vi "Traffic_Light_Simulation (1).vi"() -> ()   [LabVIEW 2020]
panel:
  out "Green 13":bool
  out "Green 11":bool
  out "Green 14":bool
  out "Green 12":bool
  out "Green 10":bool
  out "Green 9":bool
  out "Green 8":bool
  out "Green 7":bool
  out "Boolean 3":bool
  out "Yellow5":bool
  out "Green 6":bool
  out "Red 6":bool
  out "Boolean":bool
  out "Boolean 5":bool
  out "Boolean 4":bool
  out "Boolean 2":bool
  out "Red 5":bool
  out "Green 5":bool
  out "Yellow 4":bool
  out "Green 4":bool
  out "Red 4":bool
  out "Yellow4":bool
  out "Yellow 3":bool
  out "Green 3":bool
  out "Red 3":bool
  out "Red 2":bool
  out "Yellow 2":bool
  out "Green 2":bool
  in  "stop":bool
  # "|\n|\n|\n|\n|\n|\n|\n|\n|\n|\n|"
  # "Pedesterian Signal"
  # "Pedesterian Signal"
  # "Zebra Crossing"
  # "| | | | | | | | | | | | | | | | | | | | | | | | | | | | | |"
  # "Left Light"
  # "| |\n| |\n| |\n| |\n| |\n| |\n| |\n| |\n| |\n| |\n| |"
  # "| |\n| |\n| |\n| |\n| |\n| |\n| |\n| |\n| |\n| |\n| |"
  # "Left Light"
  # "Left Light"
  # "----------------------------------"
  # "Traffic Light Simulation"
  # "----------------------------------"
  # "Left Light"
  # "|\n|\n|\n|\n|\n|\n|\n|\n|\n|\n|"
  # "| | | | | | | | | | | | | | | | | | | | | | | | | | | | | |"
  # "Pedesterian Signal"
  # "Pedesterian Signal"
  # "Meaning of Traffic Lights"
  # "Go"
  # "Ready to Stop"
  # "Stop"
  # "Only Left Turns"
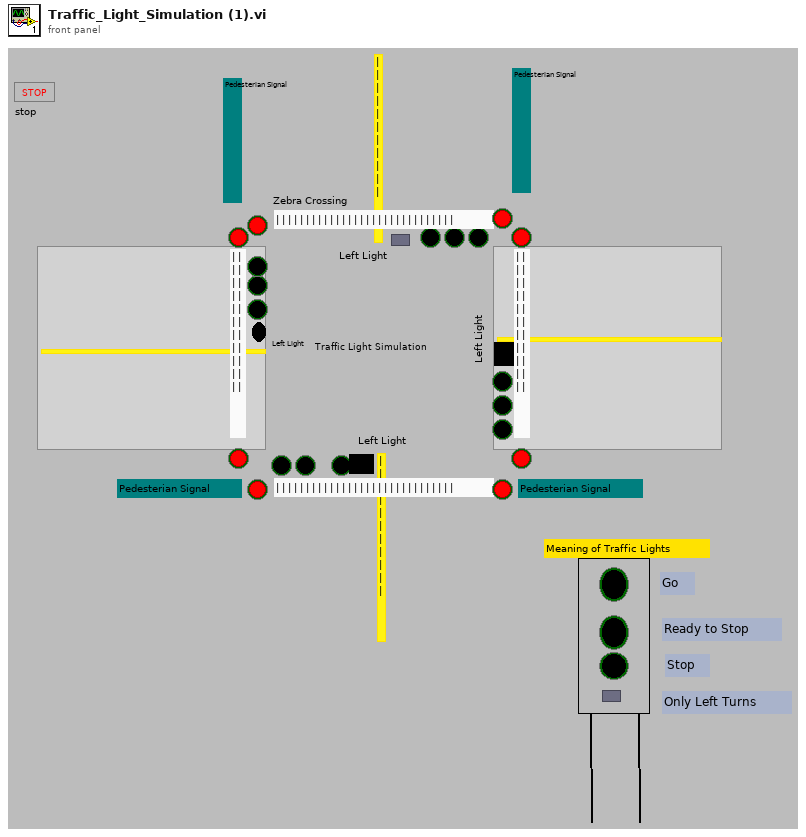
[diagram p1: front panel]
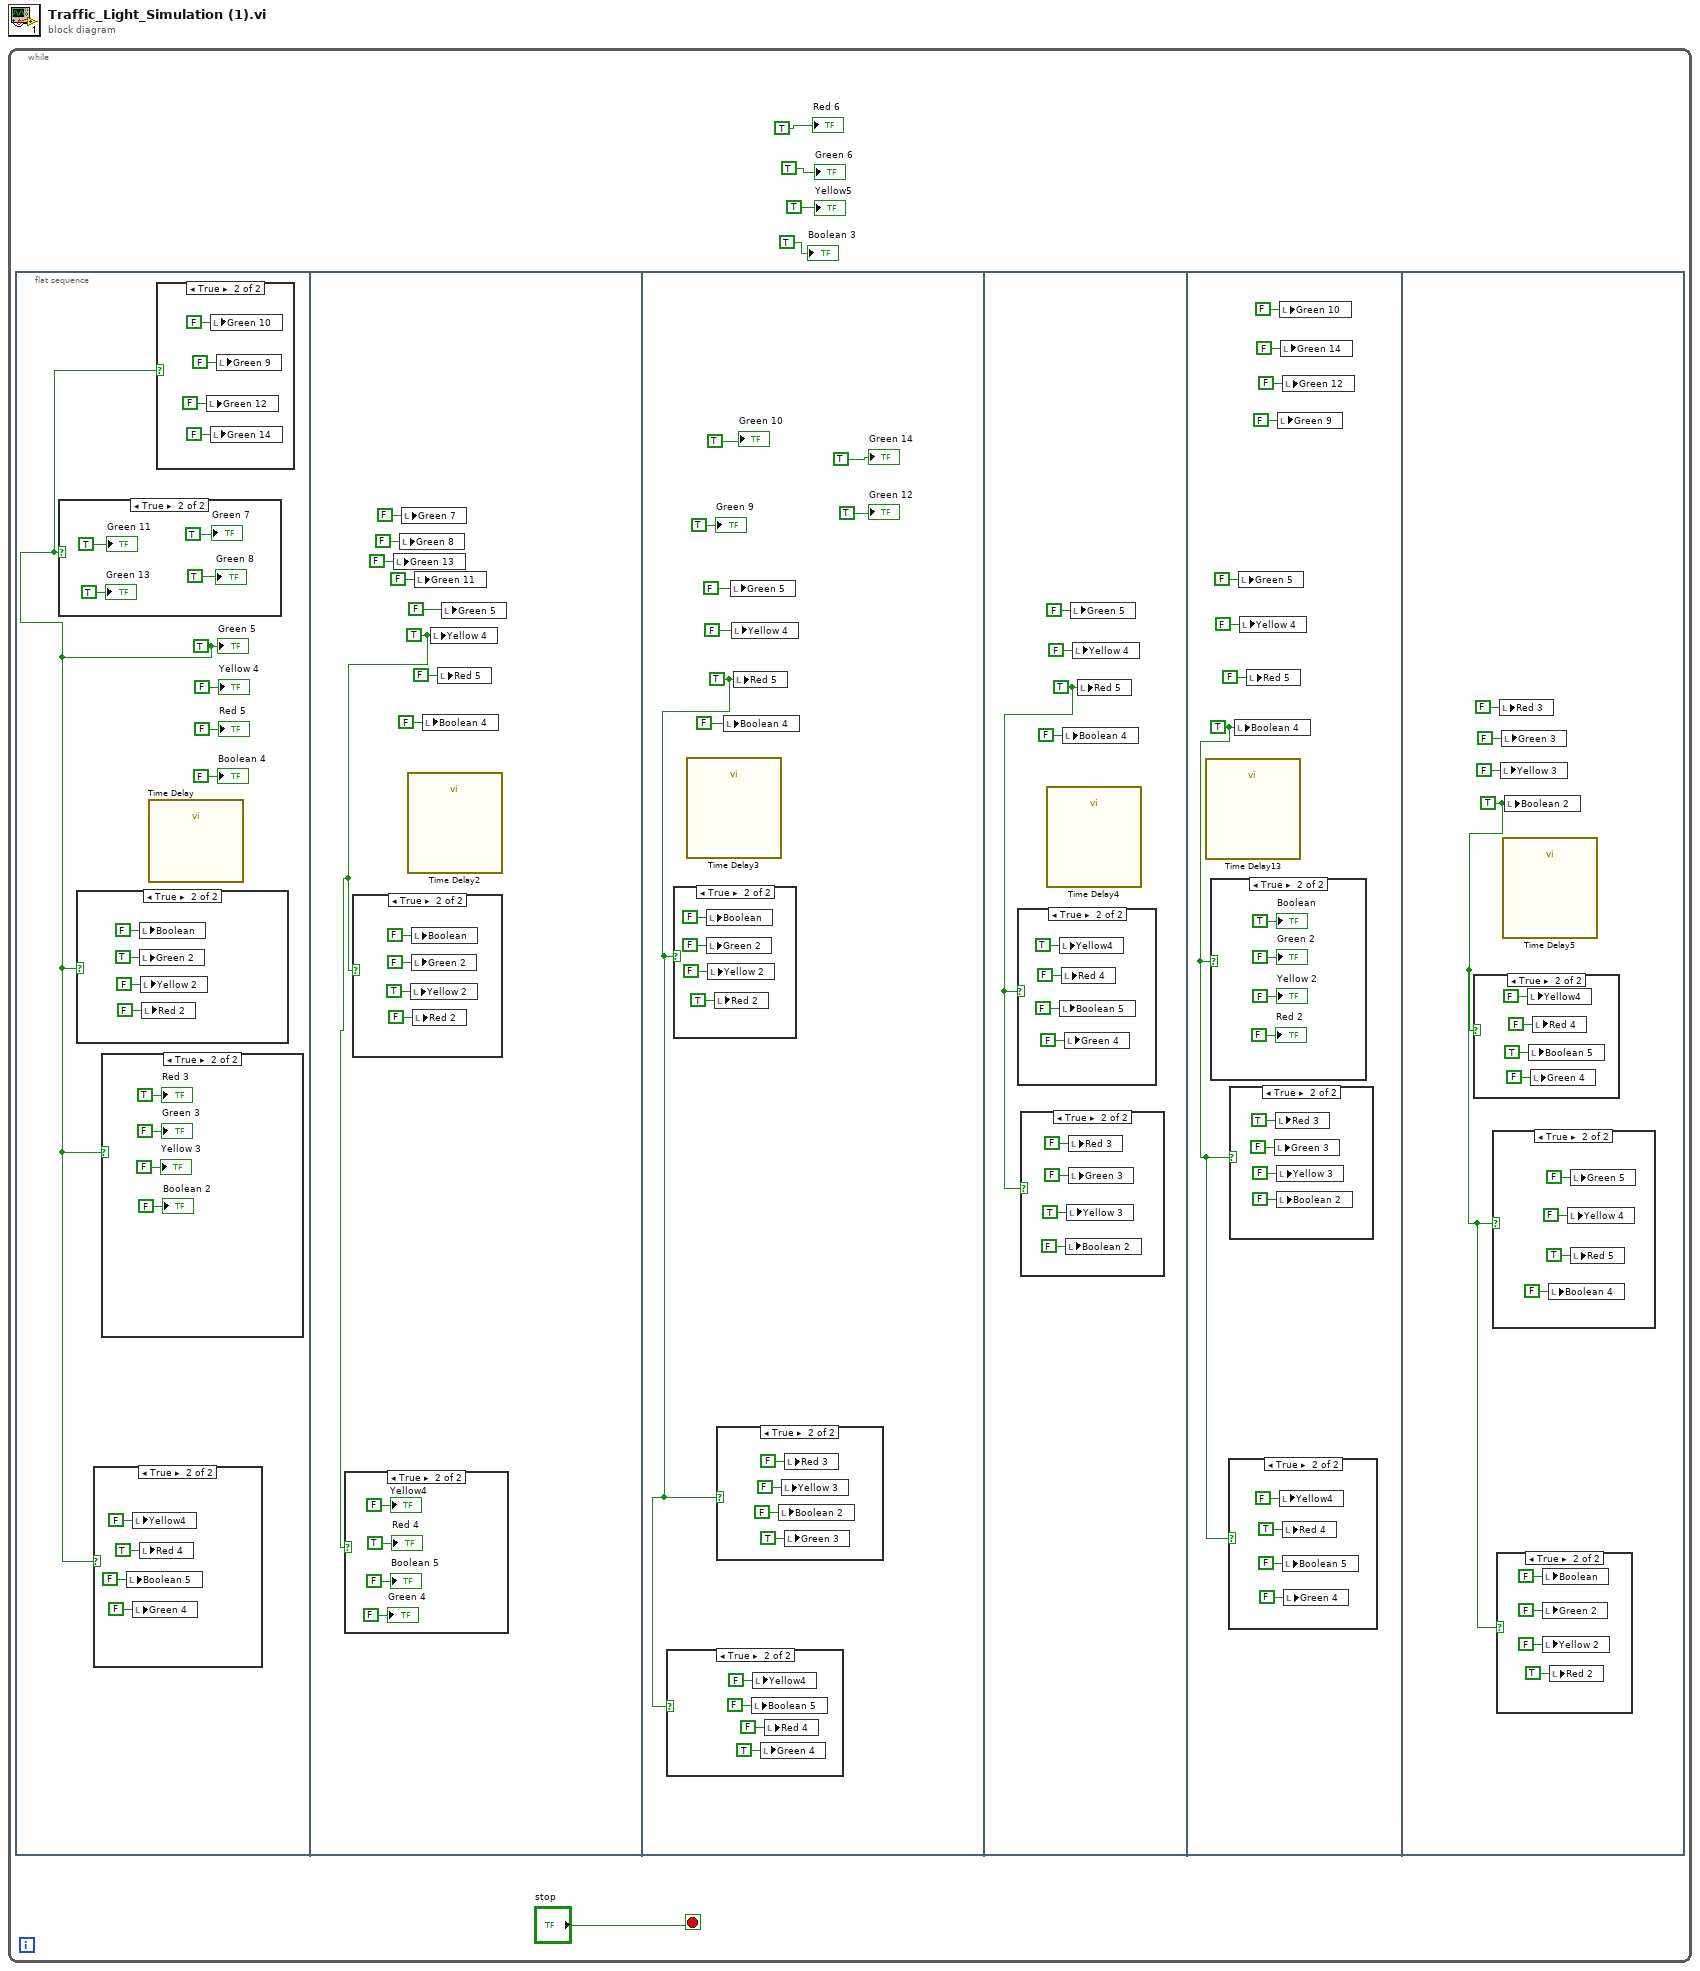
[diagram p0: block diagram]
diagram:
  n1 = while {
    stop <- "stop" stop-if-true
    n2 = flat-sequence {
      frame #0 {
        w6 = TRUE ("Green 5")
        n3 = case shown="True" w6 {
          frame False {
          }
          frame True {
            "Green 7" <- TRUE ("Green 7")
            "Green 11" <- TRUE ("Green 11")
            "Green 13" <- TRUE ("Green 13")
            "Green 8" <- TRUE ("Green 8")
          }
        }
        n4 = case shown="True" w6 {
          frame False {
          }
          frame True {
            n5 = local write "Boolean"(FALSE ("Boolean")) -> ()
            n6 = local write "Green 2"(TRUE ("Green 2")) -> ()
            n7 = local write "Yellow 2"(FALSE ("Yellow 2")) -> ()
            n8 = local write "Red 2"(FALSE ("Red 2")) -> ()
          }
        }
        n9 = case shown="True" w6 {
          frame False {
          }
          frame True {
            n10 = local write "Boolean 5"(FALSE ("Boolean 5")) -> ()
            n11 = local write "Yellow4"(FALSE ("Yellow4")) -> ()
            n12 = local write "Green 4"(FALSE ("Green 4")) -> ()
            n13 = local write "Red 4"(TRUE ("Red 4")) -> ()
          }
        }
        n14 = case shown="True" w6 {
          frame False {
          }
          frame True {
            "Red 3" <- TRUE ("Red 3")
            "Green 3" <- FALSE ("Green 3")
            "Yellow 3" <- FALSE ("Yellow 3")
            "Boolean 2" <- FALSE ("Boolean 2")
          }
        }
        n15 = call "Time Delay"() -> ()  [unwired: 11 in, 1 out]
        n16 = case shown="True" w6 {
          frame False {
          }
          frame True {
            n17 = local write "Green 12"(FALSE ("Green 12")) -> ()
            n18 = local write "Green 10"(FALSE ("Green 10")) -> ()
            n19 = local write "Green 14"(FALSE ("Green 14")) -> ()
            n20 = local write "Green 9"(FALSE ("Green 9")) -> ()
          }
        }
        "Yellow 4" <- FALSE ("Yellow 4")
        "Green 5" <- w6
        "Red 5" <- FALSE ("Red 5")
        "Boolean 4" <- FALSE ("Boolean 4")
      }
      frame #1 {
        w34 = TRUE ("Yellow 4")
        n21 = case shown="True" w34 {
          frame False {
          }
          frame True {
            "Yellow4" <- FALSE ("Yellow4")
            "Red 4" <- TRUE ("Red 4")
            "Boolean 5" <- FALSE ("Boolean 5")
            "Green 4" <- FALSE ("Green 4")
          }
        }
        n22 = case shown="True" w34 {
          frame False {
          }
          frame True {
            n23 = local write "Yellow 2"(TRUE ("Yellow 2")) -> ()
            n24 = local write "Boolean"(FALSE ("Boolean")) -> ()
            n25 = local write "Green 2"(FALSE ("Green 2")) -> ()
            n26 = local write "Red 2"(FALSE ("Red 2")) -> ()
          }
        }
        n27 = local write "Green 13"(FALSE ("Green 13")) -> ()
        n28 = local write "Green 8"(FALSE ("Green 8")) -> ()
        n29 = local write "Green 7"(FALSE ("Green 7")) -> ()
        n30 = call "Time Delay2"() -> ()  [unwired: 11 in, 1 out]
        n31 = local write "Green 11"(FALSE ("Green 11")) -> ()
        n32 = local write "Boolean 4"(FALSE ("Boolean 4")) -> ()
        n33 = local write "Yellow 4"(w34) -> ()
        n34 = local write "Red 5"(FALSE ("Red 5")) -> ()
        n35 = local write "Green 5"(FALSE ("Green 5")) -> ()
      }
      frame #2 {
        w50 = TRUE ("Red 5")
        n36 = case shown="True" w50 {
          frame False {
          }
          frame True {
            n37 = local write "Boolean 5"(FALSE ("Boolean 5")) -> ()
            n38 = local write "Yellow4"(FALSE ("Yellow4")) -> ()
            n39 = local write "Green 4"(TRUE ("Green 4")) -> ()
            n40 = local write "Red 4"(FALSE ("Red 4")) -> ()
          }
        }
        n41 = case shown="True" w50 {
          frame False {
          }
          frame True {
            n42 = local write "Boolean"(FALSE ("Boolean")) -> ()
            n43 = local write "Green 2"(FALSE ("Green 2")) -> ()
            n44 = local write "Yellow 2"(FALSE ("Yellow 2")) -> ()
            n45 = local write "Red 2"(TRUE ("Red 2")) -> ()
          }
        }
        n46 = call "Time Delay3"() -> ()  [unwired: 11 in, 1 out]
        n47 = case shown="True" w50 {
          frame False {
          }
          frame True {
            n48 = local write "Boolean 2"(FALSE ("Boolean 2")) -> ()
            n49 = local write "Yellow 3"(FALSE ("Yellow 3")) -> ()
            n50 = local write "Red 3"(FALSE ("Red 3")) -> ()
            n51 = local write "Green 3"(TRUE ("Green 3")) -> ()
          }
        }
        n52 = local write "Boolean 4"(FALSE ("Boolean 4")) -> ()
        n53 = local write "Green 5"(FALSE ("Green 5")) -> ()
        n54 = local write "Yellow 4"(FALSE ("Yellow 4")) -> ()
        n55 = local write "Red 5"(w50) -> ()
        "Green 14" <- TRUE ("Green 14")
        "Green 10" <- TRUE ("Green 10")
        "Green 9" <- TRUE ("Green 9")
        "Green 12" <- TRUE ("Green 12")
      }
      frame #3 {
        w66 = TRUE ("Red 5")
        n56 = case shown="True" w66 {
          frame False {
          }
          frame True {
            n57 = local write "Yellow4"(TRUE ("Yellow4")) -> ()
            n58 = local write "Boolean 5"(FALSE ("Boolean 5")) -> ()
            n59 = local write "Red 4"(FALSE ("Red 4")) -> ()
            n60 = local write "Green 4"(FALSE ("Green 4")) -> ()
          }
        }
        n61 = case shown="True" w66 {
          frame False {
          }
          frame True {
            n62 = local write "Boolean 2"(FALSE ("Boolean 2")) -> ()
            n63 = local write "Yellow 3"(TRUE ("Yellow 3")) -> ()
            n64 = local write "Red 3"(FALSE ("Red 3")) -> ()
            n65 = local write "Green 3"(FALSE ("Green 3")) -> ()
          }
        }
        n66 = call "Time Delay4"() -> ()  [unwired: 11 in, 1 out]
        n67 = local write "Boolean 4"(FALSE ("Boolean 4")) -> ()
        n68 = local write "Green 5"(FALSE ("Green 5")) -> ()
        n69 = local write "Yellow 4"(FALSE ("Yellow 4")) -> ()
        n70 = local write "Red 5"(w66) -> ()
      }
      frame #4 {
        w82 = TRUE ("Boolean 4")
        n71 = call "Time Delay13"() -> ()  [unwired: 11 in, 1 out]
        n72 = case shown="True" w82 {
          frame False {
          }
          frame True {
            "Boolean" <- TRUE ("Boolean")
            "Green 2" <- FALSE ("Green 2")
            "Red 2" <- FALSE ("Red 2")
            "Yellow 2" <- FALSE ("Yellow 2")
          }
        }
        n73 = case shown="True" w82 {
          frame False {
          }
          frame True {
            n74 = local write "Yellow4"(FALSE ("Yellow4")) -> ()
            n75 = local write "Red 4"(TRUE ("Red 4")) -> ()
            n76 = local write "Boolean 5"(FALSE ("Boolean 5")) -> ()
            n77 = local write "Green 4"(FALSE ("Green 4")) -> ()
          }
        }
        n78 = case shown="True" w82 {
          frame False {
          }
          frame True {
            n79 = local write "Green 3"(FALSE ("Green 3")) -> ()
            n80 = local write "Red 3"(TRUE ("Red 3")) -> ()
            n81 = local write "Yellow 3"(FALSE ("Yellow 3")) -> ()
            n82 = local write "Boolean 2"(FALSE ("Boolean 2")) -> ()
          }
        }
        n83 = local write "Boolean 4"(w82) -> ()
        n84 = local write "Green 5"(FALSE ("Green 5")) -> ()
        n85 = local write "Yellow 4"(FALSE ("Yellow 4")) -> ()
        n86 = local write "Red 5"(FALSE ("Red 5")) -> ()
        n87 = local write "Green 9"(FALSE ("Green 9")) -> ()
        n88 = local write "Green 10"(FALSE ("Green 10")) -> ()
        n89 = local write "Green 14"(FALSE ("Green 14")) -> ()
        n90 = local write "Green 12"(FALSE ("Green 12")) -> ()
      }
      frame #5 {
        w98 = TRUE ("Boolean 2")
        n91 = case shown="True" w98 {
          frame False {
          }
          frame True {
            n92 = local write "Yellow4"(FALSE ("Yellow4")) -> ()
            n93 = local write "Boolean 5"(TRUE ("Boolean 5")) -> ()
            n94 = local write "Green 4"(FALSE ("Green 4")) -> ()
            n95 = local write "Red 4"(FALSE ("Red 4")) -> ()
          }
        }
        n96 = case shown="True" w98 {
          frame False {
          }
          frame True {
            n97 = local write "Boolean 4"(FALSE ("Boolean 4")) -> ()
            n98 = local write "Yellow 4"(FALSE ("Yellow 4")) -> ()
            n99 = local write "Green 5"(FALSE ("Green 5")) -> ()
            n100 = local write "Red 5"(TRUE ("Red 5")) -> ()
          }
        }
        n101 = case shown="True" w98 {
          frame False {
          }
          frame True {
            n102 = local write "Boolean"(FALSE ("Boolean")) -> ()
            n103 = local write "Green 2"(FALSE ("Green 2")) -> ()
            n104 = local write "Yellow 2"(FALSE ("Yellow 2")) -> ()
            n105 = local write "Red 2"(TRUE ("Red 2")) -> ()
          }
        }
        n106 = local write "Red 3"(FALSE ("Red 3")) -> ()
        n107 = local write "Yellow 3"(FALSE ("Yellow 3")) -> ()
        n108 = local write "Green 3"(FALSE ("Green 3")) -> ()
        n109 = call "Time Delay5"() -> ()  [unwired: 11 in, 1 out]
        n110 = local write "Boolean 2"(w98) -> ()
      }
    }
    "Red 6" <- TRUE ("Red 3")
    "Green 6" <- TRUE ("Green 3")
    "Yellow5" <- TRUE ("Yellow 3")
    "Boolean 3" <- TRUE ("Boolean 2")
  }
